vi "Keithley617_Shutdown.vi"(7 "GPIB Address String":string="27", 8 "Error In":errorcluster) -> (0 "Error Out":errorcluster)   [LabVIEW 2015, in "Keithley617.lvlib"]
uses:
  Keithley617_GPIB_Commands.ctl
  Keithley617.lvlib
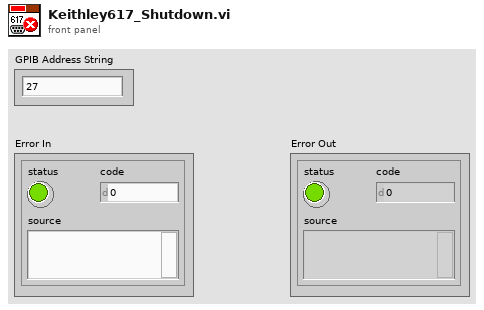
[diagram p1: front panel]
types:
  T1 = typedef "Keithley617_GPIB_Commands.ctl" = string
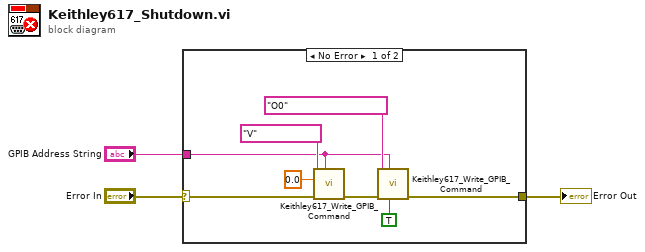
[diagram p0: block diagram]
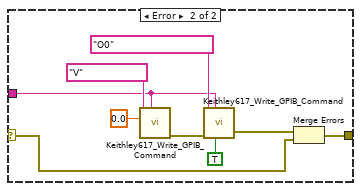
[diagram p2: hidden frame]
diagram:
  n1 = case shown="No Error" "Error In" {
    selector: "Error In" -> [w6 w14]
    tunnel: [w7 w12] -> w2
    tunnel: "GPIB Address String" -> [w4 w15]
    frame No Error {
      n2 = call "Keithley617_Write_GPIB_Command.vi"("GPIB Address String"=w4, "Error In"=w6, "Value"=0.0, "Command"=T1 "V") -> ("Error Out"=w9:errorcluster)  [unwired: 7 in]
      n3 = call "Keithley617_Write_GPIB_Command.vi"("Execute Command?"=TRUE, "GPIB Address String"=w4, "Error In"=w9, "Command"=T1 "O0") -> ("Error Out"=w7:errorcluster)  [unwired: 7 in]
    }
    frame Error {
      n4 = call "Keithley617_Write_GPIB_Command.vi"("GPIB Address String"=w15, "Value"=0.0, "Command"=T1 "V") -> ("Error Out"=w18:errorcluster)  [unwired: 8 in]
      n5 = call "Keithley617_Write_GPIB_Command.vi"("Execute Command?"=TRUE, "GPIB Address String"=w15, "Error In"=w18, "Command"=T1 "O0") -> ("Error Out"=w13:errorcluster)  [unwired: 7 in]
      n6 = Merge Errors(w13, w14) -> (w12:errorcluster)
    }
  }
  "Error Out" <- w2
